vi "Create.vi"(0 "ID":i32=-1, 5 "Object ID":i32=-1, 7 "Key":string, 9 "Value":variant, 11 "error in (no error)":errorcluster) -> (4 "Attribute out":refnum<class "Attribute.lvclass">, 15 "error out":errorcluster)   [LabVIEW 2019, in "HierDAL Library.lvlib" / "Models.lvlib" / "Attribute.lvclass"]
uses:
  Attribute.lvclass
  Attribute.lvclass/Attribute.ctl
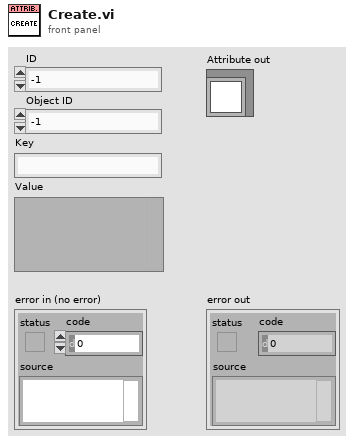
[diagram p1: front panel]
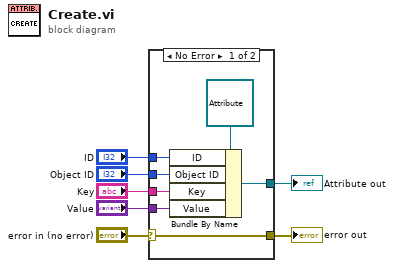
[diagram p0: block diagram]
diagram:
  n1 = case shown="No Error" "error in (no error)" {
    selector: "error in (no error)" -> [w14 w15]
    tunnel: [w14 w15] -> w6
    tunnel: "ID" -> [w9 _]
    tunnel: "Object ID" -> [w10 _]
    tunnel: "Key" -> [w11 _]
    tunnel: "Value" -> [w12 _]
    tunnel: [w8 _] -> w1
    frame No Error {
      n2 = Bundle By Name(cluster=refnum<class "Attribute.lvclass"> refnum ("Attribute out"), "ID"=w9, "Object ID"=w10, "Key"=w11, "Value"=w12) -> (w8:refnum<class "Attribute.lvclass">)
    }
    frame Error {
    }
  }
  "error out" <- w6
  "Attribute out" <- w1
